vi "曲线判定demo.vi"() -> ()   [LabVIEW 2019]
panel:
  out "OK？":bool
  in  "Result":string[][](table)
  out "XY图":cluster{dbl[], dbl[]}[](graph)
  in  "文件路径输入控件":path
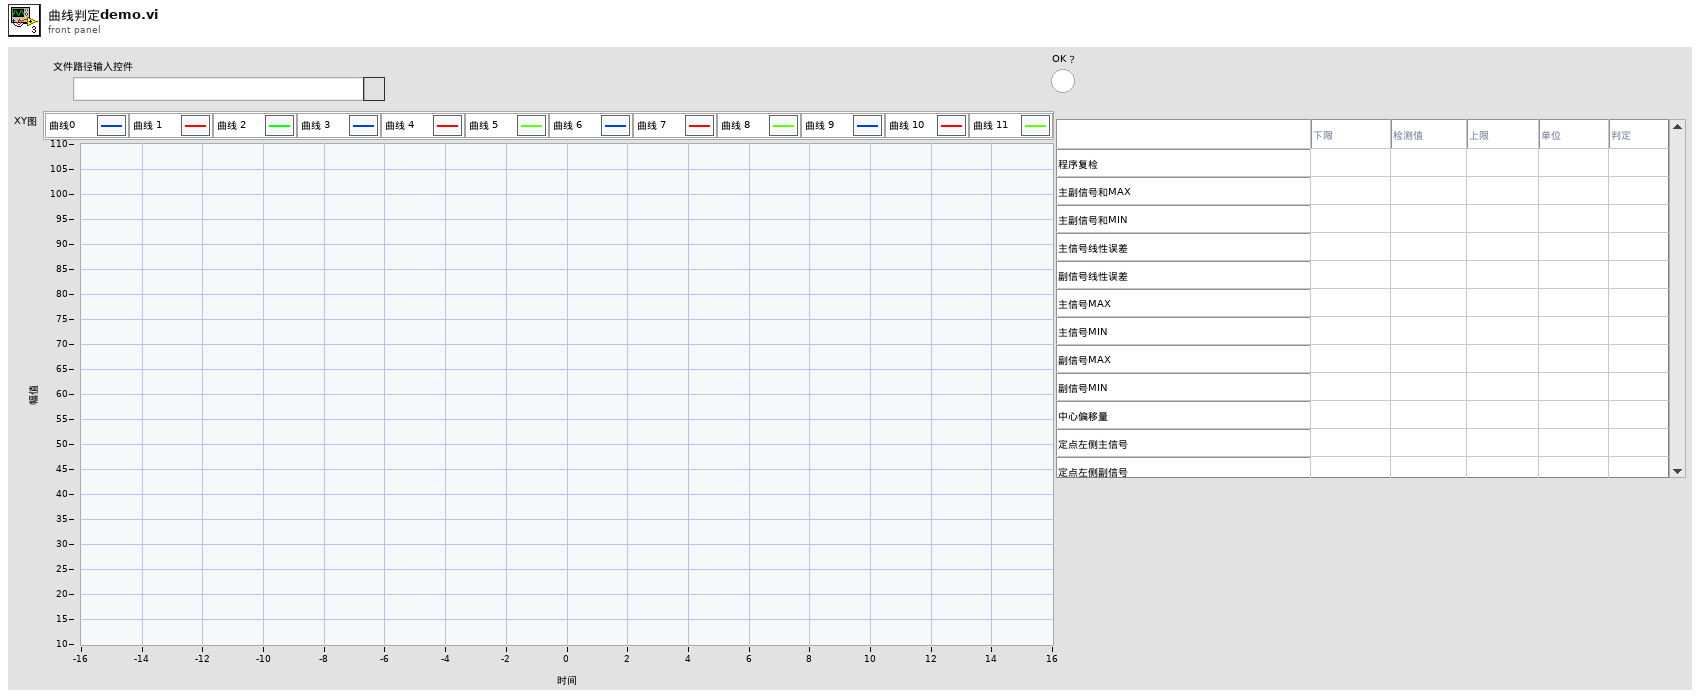
[diagram p1: front panel]
types:
  T1 = cluster{"主副信号和MAX":cluster{"单位":string, "下限":dbl, "上限":dbl}, "主副信号和MIN":cluster{"单位":string, "下限":dbl, "上限":dbl}, "主信号线性误差":cluster{"单位":string, "下限":dbl, "上限":dbl}, "副信号线性误差":cluster{"单位":string, "下限":dbl, "上限":dbl}, "主信号MAX":cluster{"单位":string, "下限":dbl, "上限":dbl}, "主信号MIN":cluster{"单位":string, "下限":dbl, "上限":dbl}, "副信号MAX":cluster{"单位":string, "下限":dbl, "上限":dbl}, "副信号MIN":cluster{"单位":string, "下限":dbl, "上限":dbl}, "中心偏移量":cluster{"单位":string, "下限":dbl, "上限":dbl}, "定点设置":cluster{"单位":string, "下限":dbl, "上限":dbl}, "定点左侧主信号":cluster{"单位":string, "下限":dbl, "上限":dbl}, "定点左侧副信号":cluster{"单位":string, "下限":dbl, "上限":dbl}, "定点右侧主信号":cluster{"单位":string, "下限":dbl, "上限":dbl}, "定点右侧副信号":cluster{"单位":string, "下限":dbl, "上限":dbl}}
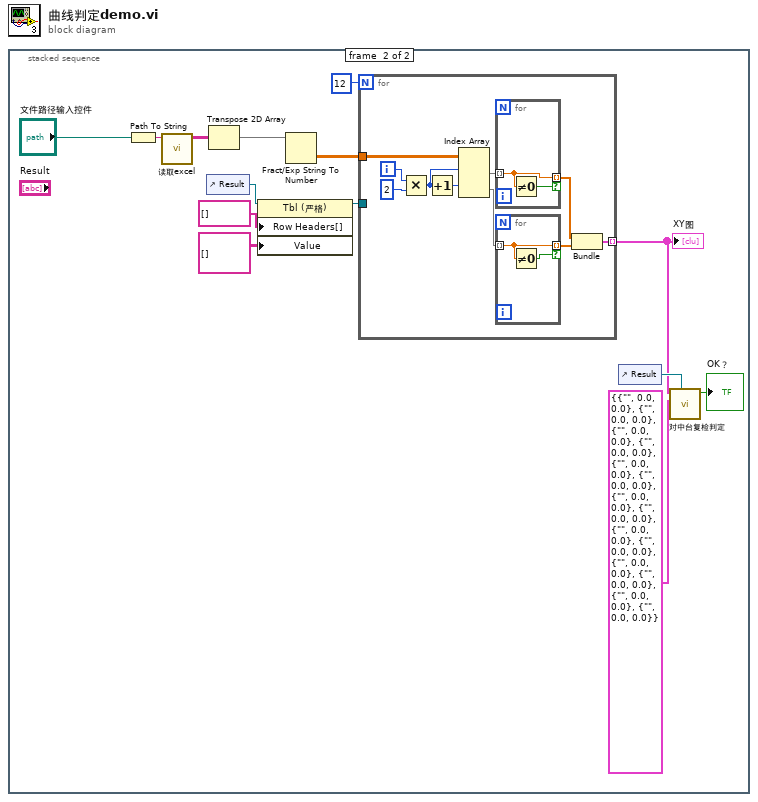
[diagram p0: block diagram]
diagram:
  n1 = stacked-sequence {
    frame #0 {
    }
    frame #1 {
      n2 = Path To String(path="文件路径输入控件") -> (string=w13:string)
      n3 = call "读取excel.vi"("Filename"=w13) -> ("数据"=w12:string[][])  [unwired: 10 in]
      n4 = control-ref of="Result"() -> (w2:refnum<vi>)
      n5 = Transpose 2D Array(2D array=w12) -> (transposed array=w11:string[][])
      n6 = property class="Tbl (严格)"(reference=w2, "Row Headers[]"=string[] [] ("行首字符串[]"), "Value"=string[][] [] ("值")) -> (reference out=w1:refnum<vi>)  [unwired: 1 in, 1 out]
      n7 = Fract/Exp String To Number(string=w11) -> (number=w10:dbl[][])  [unwired: 3 in, 1 out]
      n8 = for {
        N: 12 -> [_]
        tunnel: w10 -> [w24]
        tunnel: [w18] -> w7 mode=indexing
        tunnel: w1 -> [_]
        i -> [w22]
        n9 = Multiply(x=w22, y=2) -> (x*y=w17:i32)
        n10 = Increment(x=w17) -> (x+1=w16:i32)
        n11 = Index Array(array=w24, index (row) #1=w17, index (row) #2=w16) -> (element #1=w23:dbl[], element #2=w20:dbl[])  [unwired: 2 in]
        n12 = for {
          tunnel: w23 -> [w27] mode=indexing
          tunnel: [w27] -> w19 mode=indexing if=w28
          n13 = Not Equal To 0?(x=w27) -> (x != 0?=w28:bool)
        }
        n14 = for {
          tunnel: w20 -> [w25] mode=indexing
          tunnel: [w25] -> w15 mode=indexing if=w26
          n15 = Not Equal To 0?(x=w25) -> (x != 0?=w26:bool)
        }
        n16 = Bundle(w19, w15) -> (w18:cluster{dbl[], dbl[]})  [unwired: 1 in]
      }
      "XY图" <- w7
      n17 = control-ref of="Result"() -> (w8:refnum<vi>)
      n18 = call "对中台复检判定.vi"("Result"=w8, "判定参数"=T1 {"主副信号和MAX"={"单位"="", "下限"=0.0, "上限"=0.0}, "主副信号和MIN"={"单位"="", "下限"=0.0, "上限"=0.0}, "主信号线性误差"={"单位"="", "下限"=0.0, "上限"=0.0}, "副信号线性误差"={"单位"="", "下限"=0.0, "上限"=0.0}, "主信号MAX"={"单位"="", "下限"=0.0, "上限"=0.0}, "主信号MIN"={"单位"="", "下限"=0.0, "上限"=0.0}, "副信号MAX"={"单位"="", "下限"=0.0, "上限"=0.0}, "副信号MIN"={"单位"="", "下限"=0.0, "上限"=0.0}, "中心偏移量"={"单位"="", "下限"=0.0, "上限"=0.0}, "定点设置"={"单位"="", "下限"=0.0, "上限"=0.0}, "定点左侧主信号"={"单位"="", "下限"=0.0, "上限"=0.0}, "定点左侧副信号"={"单位"="", "下限"=0.0, "上限"=0.0}, "定点右侧主信号"={"单位"="", "下限"=0.0, "上限"=0.0}, "定点右侧副信号"={"单位"="", "下限"=0.0, "上限"=0.0}}, "XY曲线"=w7) -> ("OK？"=→"OK？":bool)  [unwired: 8 in]
    }
  }
